vi "Read Vertical Arrangement.vi"(9 "Text in":refnum<class "Text.lvclass">) -> (3 "Text out":refnum<class "Text.lvclass">, 4 "Vertical Arrangement":T1(ring))   [LabVIEW 2014, in "Text.lvclass"]
uses:
  Text.lvclass
  Text.lvclass/Text.ctl
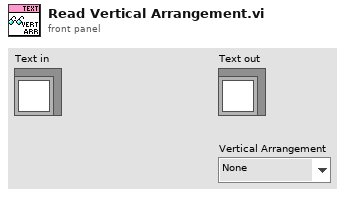
[diagram p1: front panel]
types:
  T1 = enum16{"None", "Stacked", "Clockwise", "Counterclockwise"}
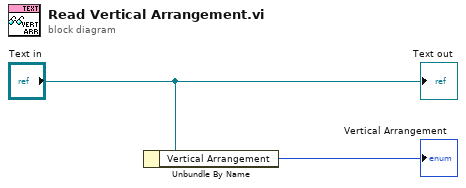
[diagram p0: block diagram]
diagram:
  n1 = Unbundle By Name("Text in") -> ("Vertical Arrangement"=→"Vertical Arrangement":T1)
  "Text out" <- "Text in"
